vi "Gen-Reader (SubVI).vi"(0 "Enum":T1, 5 "ARRAY IN":string[](array[string]), 7 "XX":string, 9 "YY":string, 11 "error in (no error)":errorcluster) -> (4 "read buffer":string, 6 "Index+1":i32, 15 "error out":errorcluster)   [LabVIEW 2014, in "CAP-USB.lvlib"]
doc: "Este VI busca el valor del elemento posterior a XX YY en el script de entrada y devuelve ese valor"
uses:
  CAP-USB.lvlib
  Enum DI-Reader.ctl
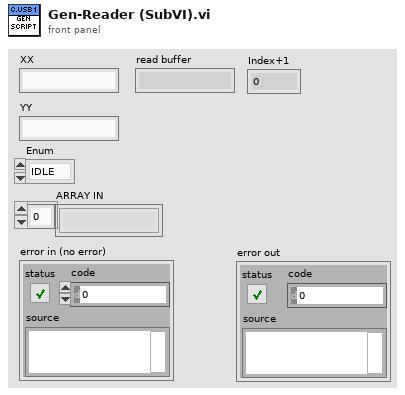
[diagram p1: front panel]
types:
  T1 = typedef "CAP-USB.lvlib/Enum DI-Reader.ctl" = enum16{"IDLE", "Detect XX", "Detect YY", "Valor", ""}
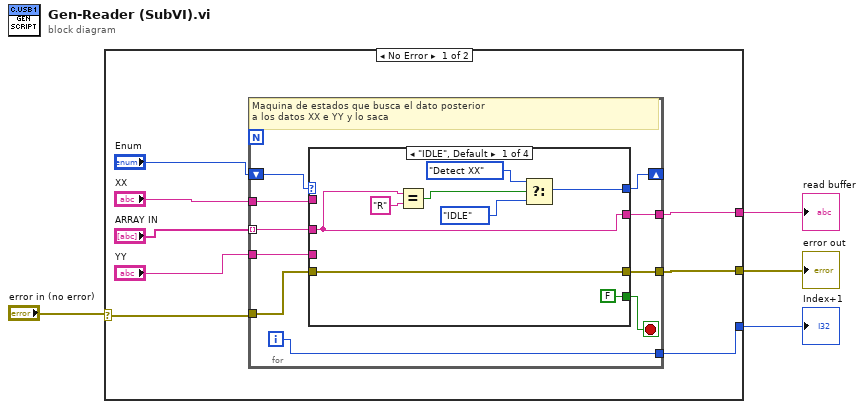
[diagram p0: block diagram]
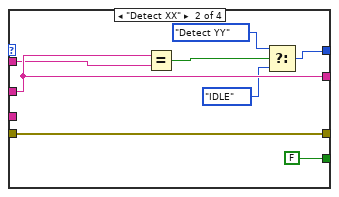
[diagram p2: hidden frame]
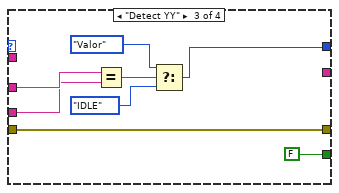
[diagram p3: hidden frame]
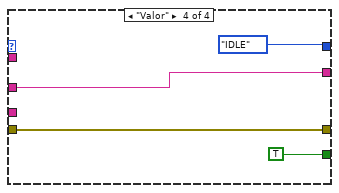
[diagram p4: hidden frame]
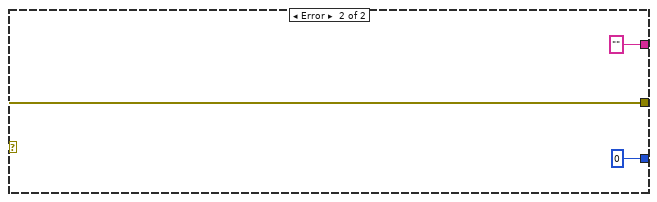
[diagram p5: hidden frame]
diagram:
  n1 = case shown="No Error" "error in (no error)" {
    selector: "error in (no error)" -> [w5 w53]
    tunnel: [w8 w53] -> w4
    tunnel: [w7 "" ("read buffer")] -> w3
    tunnel: [w6 0] -> w2
    frame No Error {
      n2 = for {
        tunnel: w5 -> [w20]
        tunnel: [w21] -> w7
        tunnel: [w22] -> w8
        tunnel: "ARRAY IN" -> [w19] mode=indexing
        shift-right: [w17] -> _
        shift-left: "Enum" -> [w18]
        tunnel: "XX" -> [w16]
        tunnel: "YY" -> [w15]
        tunnel: [w14] -> w6
        i -> [w14]
        stop <- w13 stop-if-true
        # "Maquina de estados que busca el dato posterior\na los datos XX e YY y lo saca"
        n3 = case shown="\"IDLE\", Default" w18 {
          tunnel: [w28 w37 w45 Enum_DI-Reader."IDLE"] -> w17
          tunnel: [w26 w35 _ w49] -> w21
          tunnel: [w27 w36 w44 w50] -> w22
          tunnel: w20 -> [w27 w36 w44 w50]
          tunnel: w19 -> [w26 w35 w43 w49]
          tunnel: [FALSE FALSE FALSE TRUE] -> w13
          tunnel: w15 -> [_ _ w39 _]
          tunnel: w16 -> [_ w31 _ _]
          frame "IDLE", Default {
            n4 = Equal?(x=w26, y="R") -> (x = y?=w29:bool)
            n5 = Select(t=Enum_DI-Reader."Detect XX", s=w29, f=Enum_DI-Reader."IDLE") -> (s? t:f=w28:T1)
          }
          frame "Detect XX" {
            n6 = Equal?(x=w35, y=w31) -> (x = y?=w38:bool)
            n7 = Select(t=Enum_DI-Reader."Detect YY", s=w38, f=Enum_DI-Reader."IDLE") -> (s? t:f=w37:T1)
          }
          frame "Detect YY" {
            n8 = Equal?(x=w43, y=w39) -> (x = y?=w46:bool)
            n9 = Select(t=Enum_DI-Reader."Valor", s=w46, f=Enum_DI-Reader."IDLE") -> (s? t:f=w45:T1)
          }
          frame "Valor" {
          }
        }
      }
    }
    frame Error {
    }
  }
  "error out" <- w4
  "read buffer" <- w3
  "Index+1" <- w2
